vi "Random Number (Range) DBL.vi"(10 "lower bound (0)":dbl, 11 "upper bound (100)":dbl=100.0) -> (3 "number":dbl)   [LabVIEW 2024]
doc: "<p>Generates a random value from a specified range. Wire data to the <strong>upper bound</strong> or <strong>lower bound</strong> input to determine the polymorphic instance to use or <a href=\"nihelplauncher://docs/csh?context=lvcore_lvhowto_selectingdefaultinstpolyvi\">manually select</a> the instance.</p>"
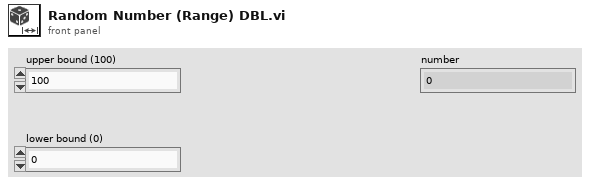
[diagram p1: front panel]
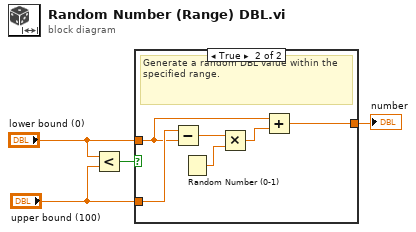
[diagram p0: block diagram]
diagram:
  n1 = Less?(x="lower bound (0)", y="upper bound (100)") -> (x < y?=w4:bool)
  n2 = case shown="True" w4 {
    tunnel: "lower bound (0)" -> [w5 w8]
    tunnel: "upper bound (100)" -> [_ w11]
    tunnel: [w5 w6] -> w1
    frame False {
      # "If bounds are reversed, always return the lower bound."
    }
    frame True {
      # "Generate a random DBL value within the specified range."
      n3 = Subtract(x=w11, y=w8) -> (x-y=w10:dbl)
      n4 = Random Number (0-1)() -> (number: 0 to 1=w9:dbl)
      n5 = Multiply(x=w10, y=w9) -> (x*y=w7:dbl)
      n6 = Add(x=w8, y=w7) -> (x+y=w6:dbl)
    }
  }
  "number" <- w1
